vi "Write Wash Display Console.vi"(8 "error in (no error)":errorcluster, 10 "Wash Display Console.lvlib:Wash Display Console.lvclass":refnum<class "Wash Display Console.lvclass">, 11 "Simulation Interface in":refnum<class "Simulation Interface.lvclass">) -> (0 "error out":errorcluster, 3 "Simulation Interface out":refnum<class "Simulation Interface.lvclass">)   [LabVIEW 2012, in "Simulation Interface.lvclass"]
uses:
  Simulation Interface.lvclass
  Wash Display Console/Wash Display Console.lvclass
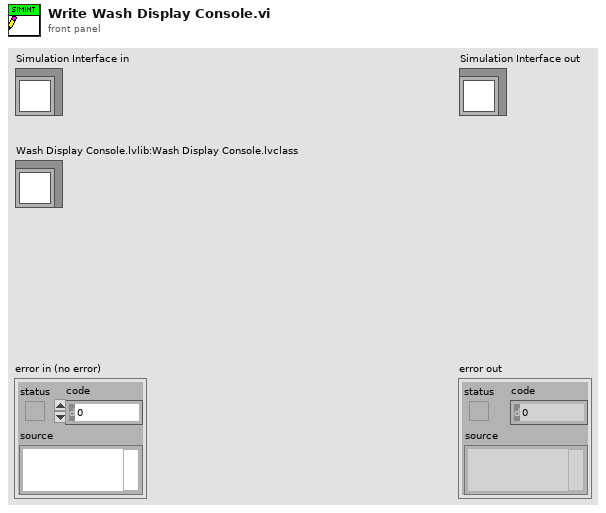
[diagram p1: front panel]
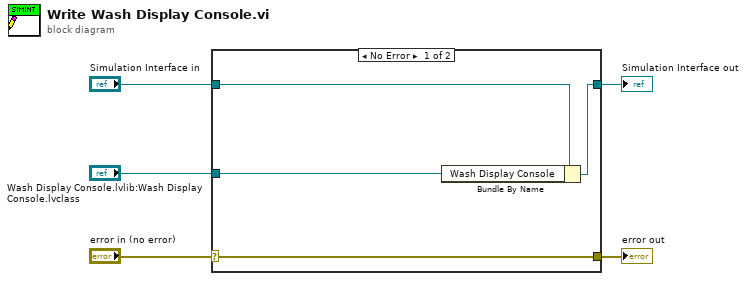
[diagram p0: block diagram]
diagram:
  n1 = case shown="No Error" "error in (no error)" {
    selector: "error in (no error)" -> [w9 w10]
    tunnel: [w9 w10] -> w4
    tunnel: [w7 w11] -> w2
    tunnel: "Simulation Interface in" -> [w8 w11]
    tunnel: "Wash Display Console.lvlib:Wash Display Console.lvclass" -> [w6 _]
    frame No Error {
      n2 = Bundle By Name(cluster=w8, "Wash Display Console"=w6) -> (w7:refnum<class "Simulation Interface.lvclass">)
    }
    frame Error {
    }
  }
  "error out" <- w4
  "Simulation Interface out" <- w2
